vi "Init Runtime.vi"(8 "error in (no error)":errorcluster, 10 "data allocations":T1, 11 "Wait On Integer Step Config in":refnum<class "Wait On Integer Config.lvclass">) -> (0 "error out":errorcluster, 2 "Skip":bool, 3 "Wait On Integer Step Config out":refnum<class "Wait On Integer Config.lvclass">)   [LabVIEW 2015, in "Wait On Integer Config.lvclass"]
uses:
  Wait On Integer Config.lvclass
  <vilib>/NI/Tag Bus Module Framework/channel/data tables.ctl
  <vilib>/NI/Tag Bus/dictionary/data dictionary.lvclass
  <vilib>/NI/Tag Bus/dictionary table pair.ctl
  <vilib>/NI/Tag Bus/table/data table.ctl
  classes/Step/Execution/StepState.ctl
  classes/Step/Execution/Step Status.ctl
  classes/Step/Execution/Step Flow Control.ctl
  Runtime/Wait On Integer.lvclass
  Wait On Integer Config.lvclass/Wait On Integer Config.ctl
  <vilib>/NI/Tag Bus/tag/tag descriptor.lvclass/tag descriptor.ctl
  Runtime/Wait On Integer.lvclass/Wait On Integer.ctl
  Read Wait On Integer Event.vi
  Read Timeout.vi
  Read Target Integer.vi
  Runtime/Write Channel Index.vi
  Runtime/Write Timeout (ms).vi
  Runtime/Write Target Integer.vi
  Runtime/Write Pass.vi
  Runtime/Write Timed Out.vi
  <vilib>/NI/Tag Bus/tag/read tag name.vi
  <vilib>/NI/Tag Bus/tag/read data type.vi
  <vilib>/NI/Tag Bus/dictionary/locate tag.vi
  <vilib>/NI/Tag Bus Module Framework/channel/TBM channel.lvclass
  classes/Step/Execution/Step.lvclass
  <vilib>/NI/Tag Bus/table/data table.lvlib
  <vilib>/NI/Tag Bus/tag bus.lvlib
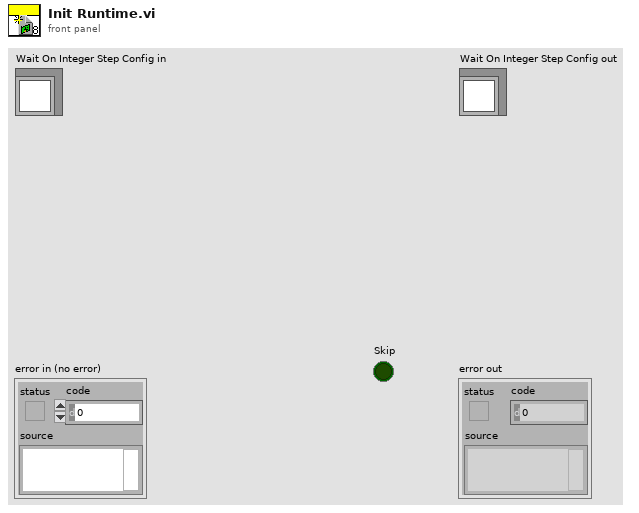
[diagram p1: front panel]
types:
  T1 = typedef "TBM channel.lvclass/data tables.ctl" = cluster{"input data":T2, "processing parameter":T2, "processing result":T2, "output data":T2}
  T2 = typedef "tag bus.lvlib/dictionary table pair.ctl" = cluster{"data dictionary":refnum<class "data dictionary.lvclass">, "data table":T3}
  T3 = typedef "tag bus.lvlib/data table.lvlib/data table.ctl" = cluster{"Double":dbl[], "Single":sgl[], "I64":i64[], "I32":i32[], "I16":i16[], "I8":i8[], "U64":u64[], "U32":u32[], "U16":u16[], "U8":u8[], "Boolean":bool[], "String":string[], "Array of Double":cluster{"DBL Array":dbl[]}[], "Array of Single":cluster{"SGL Array":sgl[]}[], "Array of I64":cluster{"I64 Array":i64[]}[], "Array of I32":cluster{"I32 Array":i32[]}[], "Array of I16":cluster{"I16 Array":i16[]}[], "Array of I8":cluster{"I8 Array":i8[]}[], "Array of U64":cluster{"U64 Array":u64[]}[], "Array of U32":cluster{"U32 Array":u32[]}[], "Array of U16":cluster{"U16 Array":u16[]}[], "Array of U8":cluster{"U8 Array":u8[]}[], "Array of Boolean":cluster{"Boolean Array":bool[]}[], "Array of String":cluster{"String Array":string[]}[]}
  T4 = typedef "Step.lvclass/StepState.ctl" = cluster{"Step State":T5, "Flow Control":T6, "Jump Index":i32, "Done":bool}
  T5 = typedef "Step.lvclass/Step Status.ctl" = enum16{"Start", "Passed", "Failed", "Error", "Done", "Terminated", "Skipped", "Running"}
  T6 = typedef "Step.lvclass/Step Flow Control.ctl" = enum16{"Next Step", "Jump"}
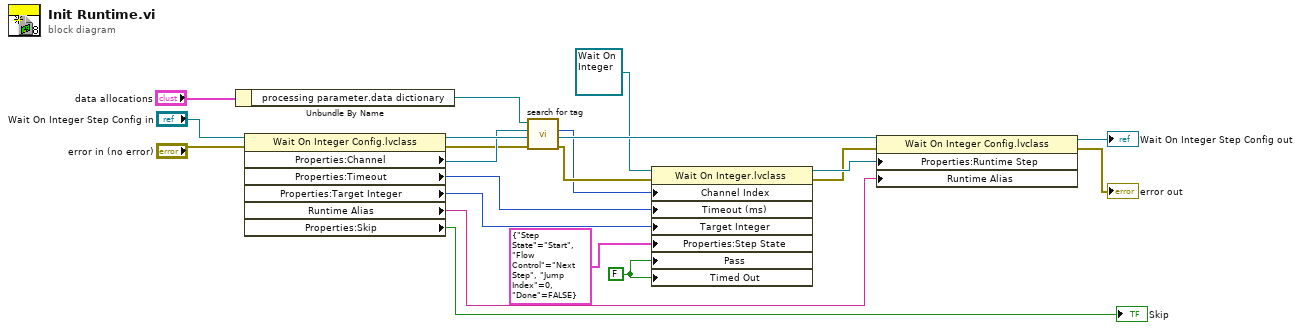
[diagram p0: block diagram]
diagram:
  w15 = FALSE ("Results")
  n1 = Unbundle By Name("data allocations") -> ("processing parameter.data dictionary"=w18:refnum<class "data dictionary.lvclass">)
  n2 = property class="Wait On Integer Config.lvclass"(reference="Wait On Integer Step Config in", error in="error in (no error)") -> (reference out=w14:refnum<class "Wait On Integer Config.lvclass">, error out=w12:errorcluster, "Properties:Channel"=w13:refnum<class "TBM channel.lvclass">, "Properties:Timeout"=w10:i32, "Properties:Target Integer"=w1:u32, "Runtime Alias"=w11:string, "Properties:Skip"=→"Skip":bool)
  n3 = call <vilib>:"search for tag.vi"("error in"=w12, "system tag"=w13, "data dictionary in"=w18) -> ("error out"=w16:errorcluster, "index"=w9:i32)  [unwired: 6 in, 1 out]
  n4 = property class="Wait On Integer.lvclass"(reference=refnum<class "Wait On Integer.lvclass"> refnum ("Wait On Integer Step.lvclass"), error in=w16, "Channel Index"=w9, "Timeout (ms)"=w10, "Target Integer"=w1, "Properties:Step State"=T4 {"Step State"=enum."Start", "Flow Control"=enum."Next Step", "Jump Index"=0, "Done"=FALSE} ("Step State"), "Pass"=w15, "Timed Out"=w15) -> (reference out=w20:refnum<class "Wait On Integer.lvclass">, error out=w19:errorcluster)
  n5 = property class="Wait On Integer Config.lvclass"(reference=w14, error in=w19, "Properties:Runtime Step"=w20, "Runtime Alias"=w11) -> (reference out=→"Wait On Integer Step Config out":refnum<class "Wait On Integer Config.lvclass">, error out=→"error out":errorcluster)
